vi "Load Config.vi"(0 "error in":errorcluster, 1 "Path":path) -> (7 "error out":errorcluster, 8 "Cluster 2":T1)   [LabVIEW 2026]
uses:
  ConfigCluster.ctl
  Config Clusters/Channel Setup/(Main) Channel Setup.ctl
  Config Clusters/Channel Setup/Channel Interfaces.ctl
  Config Clusters/Channel Setup/Micropulse.ctl
  Config Clusters/Channel Setup/Gates.ctl
  Config Clusters/Scan Setup/(Main) Scan Setup.ctl
  Config Clusters/Scan Setup/Scan Settings.ctl
  Config Clusters/Scan Setup/Scan Information.ctl
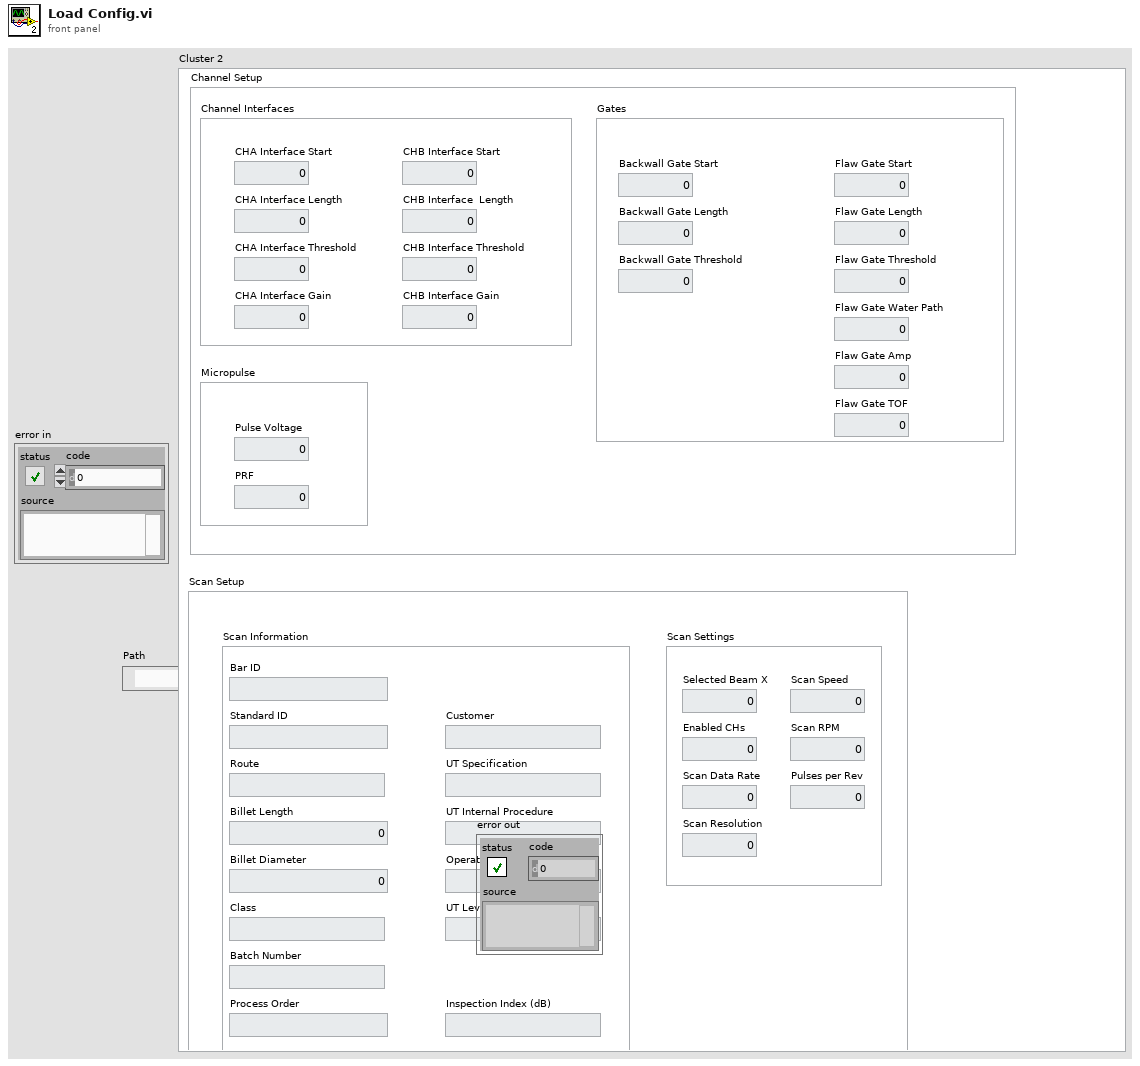
[diagram p1: front panel]
types:
  T1 = typedef "ConfigCluster.ctl" = cluster{"Channel Setup":T2, "Scan Setup":T6}
  T2 = typedef "(Main) Channel Setup.ctl" = cluster{"Channel Interfaces":T3, "Micropulse":T4, "Gates":T5}
  T3 = typedef "Channel Interfaces.ctl" = cluster{"CHA Interface Start":dbl, "CHA Interface Length":dbl, "CHA Interface Threshold":dbl, "CHA Interface Gain":dbl, "CHB Interface Start":dbl, "CHB Interface  Length ":dbl, "CHB Interface Threshold":dbl, "CHB Interface Gain":dbl}
  T4 = typedef "Micropulse.ctl" = cluster{"Pulse Voltage":dbl, "PRF":dbl}
  T5 = typedef "Gates.ctl" = cluster{"Backwall Gate Start":dbl, "Backwall Gate Length":dbl, "Backwall Gate Threshold":dbl, "Flaw Gate Start":dbl, "Flaw Gate Length":dbl, "Flaw Gate Threshold":dbl, "Flaw Gate Water Path":dbl, "Flaw Gate Amp":dbl, "Flaw Gate TOF":dbl}
  T6 = typedef "(Main) Scan Setup.ctl" = cluster{"Scan Settings":T7, "Scan Information":T8}
  T7 = typedef "Scan Settings.ctl" = cluster{"Selected Beam X":dbl, "Enabled CHs":dbl, "Scan Data Rate":dbl, "Scan Resolution":dbl, "Scan Speed":dbl, "Scan RPM":dbl, "Pulses per Rev":dbl}
  T8 = typedef "Scan Information.ctl" = cluster{"Bar Alloy":string, "Batch Number":string, "Class":string, "Route":string, "Customer":string, "UT Specification":string, "UT Internal Procedure":string, "Operator":string, "UT Level":string, "Inspection Index (dB)":string, "Scanname":string, "Process Order":string, "Billet Diameter":dbl, "Billet Length":dbl, "Bar ID":string, "Standard ID":string}
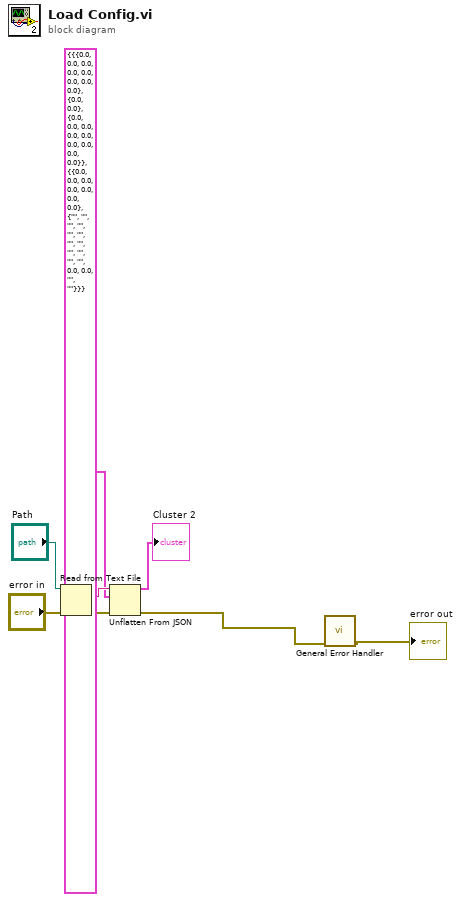
[diagram p0: block diagram]
diagram:
  n1 = Read from Text File(file (use dialog)="Path", error in="error in") -> (text=w6:string, error out=w5:errorcluster)  [unwired: 2 in, 2 out]
  n2 = Unflatten From JSON(JSON string=w6, type and defaults=T1 {"Channel Setup"={"Channel Interfaces"={"CHA Interface Start"=0.0, "CHA Interface Length"=0.0, "CHA Interface Threshold"=0.0, "CHA Interface Gain"=0.0, "CHB Interface Start"=0.0, "CHB Interface  Length "=0.0, "CHB Interface Threshold"=0.0, "CHB Interface Gain"=0.0}, "Micropulse"={"Pulse Voltage"=0.0, "PRF"=0.0}, "Gates"={"Backwall Gate Start"=0.0, "Backwall Gate Length"=0.0, "Backwall Gate Threshold"=0.0, "Flaw Gate Start"=0.0, "Flaw Gate Length"=0.0, "Flaw Gate Threshold"=0.0, "Flaw Gate Water Path"=0.0, "Flaw Gate Amp"=0.0, "Flaw Gate TOF"=0.0}}, "Scan Setup"={"Scan Settings"={"Selected Beam X"=0.0, "Enabled CHs"=0.0, "Scan Data Rate"=0.0, "Scan Resolution"=0.0, "Scan Speed"=0.0, "Scan RPM"=0.0, "Pulses per Rev"=0.0}, "Scan Information"={"Bar Alloy"="", "Batch Number"="", "Class"="", "Route"="", "Customer"="", "UT Specification"="", "UT Internal Procedure"="", "Operator"="", "UT Level"="", "Inspection Index (dB)"="", "Scanname"="", "Process Order"="", "Billet Diameter"=0.0, "Billet Length"=0.0, "Bar ID"="", "Standard ID"=""}}} ("Cluster 2"), error in (no error)=w5) -> (value=→"Cluster 2":T1, error out=w2:errorcluster)  [unwired: 4 in]
  n3 = call <vilib>:"General Error Handler.vi"("error in (no error)"=w2) -> ("error out"=→"error out":errorcluster)  [unwired: 10 in, 4 out]
